vi "NT_LL_Read Int Array.vi"(8 "error in (no error)":errorcluster, 10 "default value":i64[](array[numeric]), 11 "subscribeHandle":u32) -> (0 "error out":errorcluster, 2 "time":i64, 3 "value":i64[](array[numeric]))   [LabVIEW 2025]
uses:
  FRC_NetworkTablesLV.dll
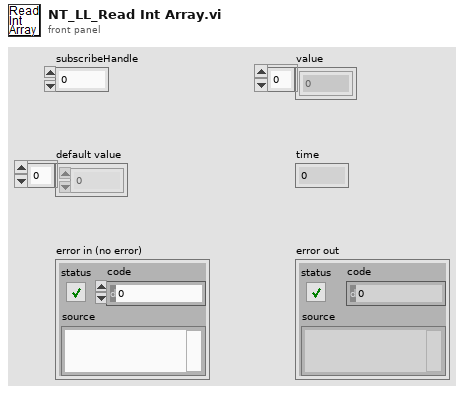
[diagram p1: front panel]
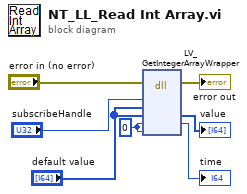
[diagram p0: block diagram]
diagram:
  w7 = i64 0 ("serverTime")
  n1 = dll-call lib="FRC_NetworkTablesLV.*" fn="LV_GetIntegerArrayWrapper"(error in="error in (no error)", "subHandle"="subscribeHandle", "defaultValue"="default value", "value"="default value", "time"=w7, "serverTime"=w7) -> (error out=→"error out":errorcluster, "value"=→"value":i64[], "time"=→"time":i64)  [unwired: 6 in, 1 out]
